vi "Address Based Construct.vi"(8 "error in":errorcluster, 9 "1553 address based handles":T1[](array[typedef]) {"acyclic frame trigger handles"."handle" format="%.0x"; "start stop handles"."stop handle" format="%.0x"; "start stop handles"."start handle" format="%.0x"}, 10 "1553 channels":T6[](array[typedef]), 11 "id":string) -> (0 "error out":errorcluster, 3 "Address Based Execution Unit Implementation out":refnum<class "Address Based Execution Unit.lvclass">)   [LabVIEW 2020, in "AIM MIL-STD-1553 Engine.lvlib" / "Implementation.lvlib" / "Address Based Execution Unit.lvclass"]
uses:
  Address Based Execution Unit.lvclass
  C:/Users/nitest/Desktop/clonetemp/Custom Device Support/Engine/Implementation/Execution Unit/Execution Unit.lvclass
  Shared/1553 Channel.ctl
  Shared/Address.ctl
  Shared/Message Definition.ctl
  Shared/Message Type.ctl
  Shared/Terminal Endpoint.ctl
  Shared/Parameter Definition.ctl
  1553 Address Based Handles.ctl
  Start Stop Channel Handles.ctl
  <vilib>/NI VeriStand/Custom Device API/Custom Device Item Ref.ctl
  Acyclic Frame Trigger Handle.ctl
  Address Based Execution Unit.lvclass/Address Based Execution Unit.ctl
  Execution Unit/Execution Unit.lvclass
  <vilib>/NI VeriStand/Custom Device API/Custom Device API.lvlib
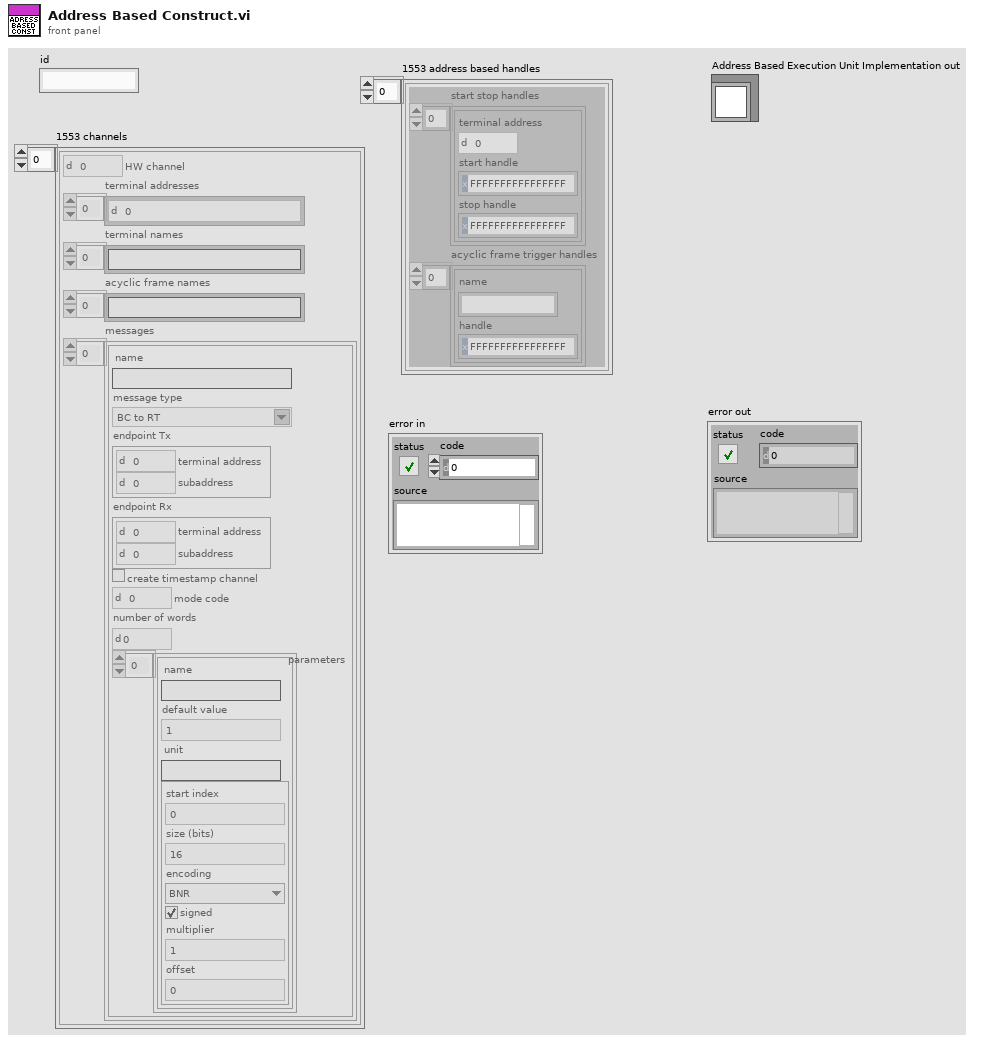
[diagram p1: front panel]
types:
  T1 = typedef "AIM MIL-STD-1553 Engine.lvlib/Implementation.lvlib/Address Based Execution Unit.lvclass/1553 Address Based Handles.ctl" = cluster{"start stop handles":T2[], "acyclic frame trigger handles":T5[]}
  T2 = typedef "AIM MIL-STD-1553 Engine.lvlib/Implementation.lvlib/Address Based Execution Unit.lvclass/Start Stop Channel Handles.ctl" = cluster{"terminal address":T3, "start handle":T4, "stop handle":T4}
  T3 = typedef "Address.ctl" = u16
  T4 = typedef "Custom Device API.lvlib/Custom Device Item Ref.ctl" = u64
  T5 = typedef "AIM MIL-STD-1553 Engine.lvlib/Implementation.lvlib/Address Based Execution Unit.lvclass/Acyclic Frame Trigger Handle.ctl" = cluster{"name":string, "handle":T4}
  T6 = typedef "1553 Channel.ctl" = cluster{"HW channel":u16, "terminal addresses":T3[], "terminal names":string[], "acyclic frame names":string[], "messages":T7[]}
  T7 = typedef "Message Definition.ctl" = cluster{"name":string, "message type":T8, "endpoint Tx":T9, "endpoint Rx":T9, "create timestamp channel":bool, "mode code":u16, "number of words":u16, "parameters":cluster{"name":string, "default value":dbl, "unit":string, "parameter definition":T10}[]}
  T8 = typedef "Message Type.ctl" = string
  T9 = typedef "Terminal Endpoint.ctl" = cluster{"terminal address":T3, "subaddress":T3}
  T10 = typedef "Parameter Definition.ctl" = cluster{"start index":i32, "size (bits)":i32, "encoding":enum16{"BNR", "BCD", "Discrete"}, "signed":bool, "multiplier":dbl, "offset":dbl}
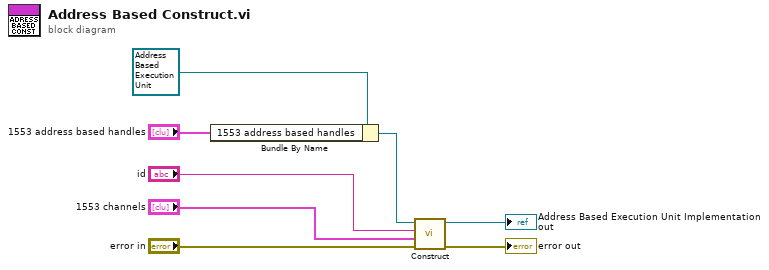
[diagram p0: block diagram]
diagram:
  n1 = Bundle By Name(cluster=refnum<class "Address Based Execution Unit.lvclass"> refnum ("Communication Bus Template Interfaces:Implementation.lvlib:Address Based Execution Unit.lvclass"), "1553 address based handles"="1553 address based handles") -> (w2:refnum<class "Address Based Execution Unit.lvclass">)
  n2 = call "Construct.vi"("error in"="error in", "1553 channels"="1553 channels", "id"="id", "Execution Unit Implementation"=w2) -> ("error out"=→"error out":errorcluster, "Execution Unit Implementation out"=→"Address Based Execution Unit Implementation out":refnum<class "Address Based Execution Unit.lvclass">)  [unwired: 6 in]
